vi "initialize Session Data.vi"(0 "OBJ - Session in":refnum<class "FPGA Session.lvclass">, 11 "error in":errorcluster) -> (4 "OBJ - Session out":refnum<class "FPGA Session.lvclass">, 15 "error out":errorcluster)   [LabVIEW 2017, in "FPGA Session.lvclass"]
doc: "OVERRIDE VI\nPlaceholder for decendant sessions to initialize and set their default values"
uses:
  FPGA Session.lvclass
  FPGA Session.lvclass/FPGA Session.ctl
  <vilib>/FPGAPlugInAG/cRIO-9081/niLvFpga_Open_cRIO-9081.vi
  <vilib>/rvi/interface/common/niFpgaWaitOnOcc.vi
  <vilib>/Utility/error.llb/Error Cluster From Error Code.vi
  <vilib>/rvi/errors/niLvFpgaAdjustHostInterfaceError.vi
  <vilib>/rvi/interface/nirviOpenFPGA/nirviOpenFPGA.xnode
  FPGA Ref.ctl
  FPGA Bitfiles/server.lvbitx
  <vilib>/rvi/interface/nirviMethod/nirviMethod.xnode
  <vilib>/rvi/interface/nirviReadWriteControl/nirviReadWriteControl.xnode
  <vilib>/rvi/errors/niLvFpgaMergeErrorWithErrorCode.vi
  <vilib>/FPGAPlugInAG/cRIO-9081/niLvFpga_ConfigureFifo_cRIO-9081.vi
  <vilib>/FPGAPlugInAG/cRIO-9081/niLvFpga_StartFifo_cRIO-9081.vi
  NiFpgaLv.dll
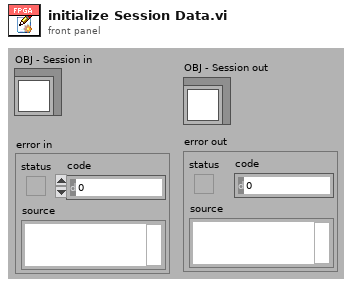
[diagram p1: front panel]
types:
  T1 = typedef "FPGA Ref.ctl" = refnum<k20>
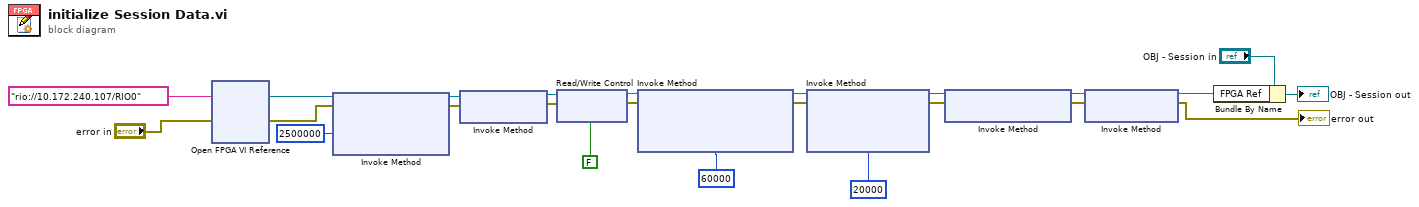
[diagram p0: block diagram]
diagram:
  n1 = xnode "Open FPGA VI Reference"("error in"="error in", "resource name"=tag "rio://10.172.240.107/RIO0") -> ("FPGA VI Reference Out"=w17:T1, "error out"=w13:errorcluster)
  n2 = xnode "Invoke Method"("FPGA VI Reference In"=w17, "error in"=w13, "Requested Depth"=u32 2500000) -> ("FPGA VI Reference Out"=w20:T1, "error out"=w19:errorcluster)  [unwired: 1 out]
  n3 = xnode "Invoke Method"("FPGA VI Reference In"=w20, "error in"=w19) -> ("FPGA VI Reference Out"=w15:T1, "error out"=w14:errorcluster)
  n4 = xnode "Read/Write Control"("FPGA VI Reference In"=w15, "error in"=w14, "Transmit?"=FALSE) -> ("FPGA VI Reference Out"=w8:T1, "error out"=w7:errorcluster)
  n5 = xnode "Invoke Method"("FPGA VI Reference In"=w8, "error in"=w7, "Requested Depth"=u32 60000) -> ("FPGA VI Reference Out"=w12:T1, "error out"=w11:errorcluster)  [unwired: 1 out]
  n6 = xnode "Invoke Method"("FPGA VI Reference In"=w12, "error in"=w11, "Requested Depth"=u32 20000) -> ("FPGA VI Reference Out"=w6:T1, "error out"=w5:errorcluster)  [unwired: 1 out]
  n7 = xnode "Invoke Method"("FPGA VI Reference In"=w6, "error in"=w5) -> ("FPGA VI Reference Out"=w4:T1, "error out"=w3:errorcluster)
  n8 = xnode "Invoke Method"("FPGA VI Reference In"=w4, "error in"=w3) -> ("FPGA VI Reference Out"=w2:T1, "error out"=→"error out":errorcluster)
  n9 = Bundle By Name(cluster="OBJ - Session in", "FPGA Ref"=w2) -> (→"OBJ - Session out":refnum<class "FPGA Session.lvclass">)
